vi "Tree.vi"   [LabVIEW 2016, in "Control Experiment.lvclass"]
uses:
  Control Experiment.lvclass
  <userlib>/LevyLab/Krohn Hite 7008/Instrument.KH7008.lvclass
  <userlib>/LevyLab/Lockin-Multichannel/Instrument.Lockin/Instrument.Lockin.lvclass
  <userlib>/LevyLab/LV to ITX/LVtoITX.lvclass
types:
  T1 = typedef "Control Experiment.lvclass/Instruments--cluster.ctl" = cluster{"KH7008":refnum<class "Instrument.KH7008.lvclass">, "Lockin":refnum<class "Instrument.Lockin.lvclass">, "Temperature":refnum<class "Instrument.Cryostat.lvclass">, "Magnet":refnum<class "Instrument.Cryostat.lvclass">, "Rotator":refnum<class "Instrument.Cryostat.lvclass">, "Level":refnum<class "Instrument.Cryostat.lvclass">}
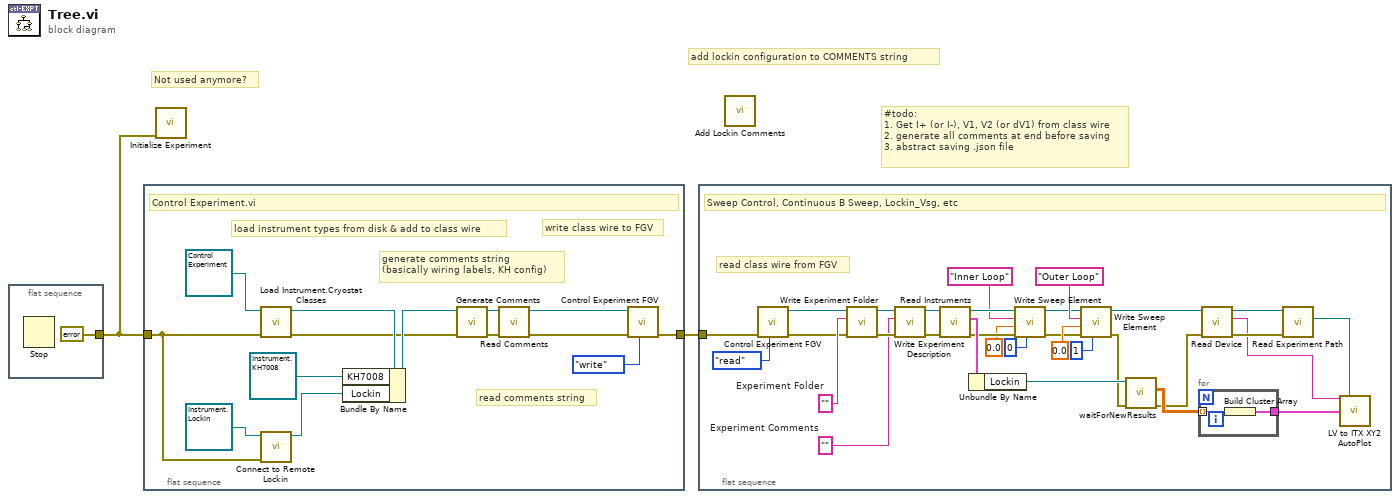
[diagram p0: block diagram]
diagram:
  # "#todo:\n1. Get I+ (or I-), V1, V2 (or dV1) from class wire\n2. generate all comments at end before saving\n3. abstract saving .json file"
  # "add lockin configuration to COMMENTS string"
  # "Not used anymore?"
  n1 = flat-sequence {
    tunnel: [errorcluster {"status"=FALSE, "code"=0, "source"=""} ("error in (no error)")] -> w2
    frame #0 {
      n2 = Stop() -> ()  [unwired: 1 in]
    }
  }
  n3 = flat-sequence {
    tunnel: w2 -> [w5]
    tunnel: [w4] -> w1
    frame #0 {
      # "write class wire to FGV"
      # "read comments string"
      # "generate comments string\n(basically wiring labels, KH config)"
      # "load instrument types from disk & add to class wire"
      # "Control Experiment.vi"
      n4 = call "Load Instrument.Cryostat Classes.vi"("error in (no error)"=w5, "Control Experiment.lvclass"=refnum<class "Control Experiment.lvclass"> refnum) -> ("error out"=w10:errorcluster, "Control Experiment out"=w12:refnum<class "Control Experiment.lvclass">)  [unwired: 8 in]
      n5 = call <userlib>:"Connect to Remote Lockin.vi"("error in (no error)"=w5, "Instrument.Lockin in"=refnum<class "Instrument.Lockin.lvclass"> refnum ("Instruments.Lockin")) -> ("Instrument.Lockin out"=w14:refnum<class "Instrument.Lockin.lvclass">)  [unwired: 8 in, 1 out]
      n6 = Bundle By Name(cluster=w12, "KH7008"=refnum<class "Instrument.KH7008.lvclass"> refnum ("Instruments.KH7008"), "Lockin"=w14) -> (w11:refnum<class "Control Experiment.lvclass">)
      n7 = call "Generate Comments.vi"("error in (no error)"=w10, "Control Experiment"=w11) -> ("error out"=w17:errorcluster, "Control Experiment out"=w16:refnum<class "Control Experiment.lvclass">)  [unwired: 7 in]
      n8 = call "Read Comments.vi"("error in (no error)"=w17, "Control Experiment in"=w16) -> ("error out"=w8:errorcluster, "Control Experiment out"=w7:refnum<class "Control Experiment.lvclass">)  [unwired: 7 in, 1 out]
      n9 = call "Control Experiment FGV.vi"("Function"=enum16{"read", "write"}."write", "error in (no error)"=w8, "Control Experiment.lvclass"=w7) -> ("error out"=w4:errorcluster)  [unwired: 7 in, 1 out]
    }
  }
  n10 = call "Initialize Experiment.vi"("error in (no error)"=w2) -> ()  [unwired: 8 in, 3 out]
  n11 = flat-sequence {
    tunnel: w1 -> [w48]
    frame #0 {
      w43 = ""  # Experiment Comments
      w44 = ""  # Experiment Folder
      # "read class wire from FGV"
      # "Sweep Control, Continuous B Sweep, Lockin_Vsg, etc"
      n12 = call "Control Experiment FGV.vi"("Function"=enum16{"read", "write"}."read", "error in (no error)"=w48) -> ("error out"=w42:errorcluster, "Control Experiment.lvclass out"=w41:refnum<class "Control Experiment.lvclass">)  [unwired: 8 in]
      n13 = call "Write Experiment Folder.vi"("error in (no error)"=w42, "Experiment Folder"=w44, "Control Experiment in"=w41) -> ("error out"=w45:errorcluster, "Control Experiment out"=w46:refnum<class "Control Experiment.lvclass">)  [unwired: 7 in]
      n14 = call "Write Experiment Description.vi"("error in (no error)"=w45, "Experiment Description"=w43, "Control Experiment in"=w46) -> ("error out"=w40:errorcluster, "Control Experiment out"=w39:refnum<class "Control Experiment.lvclass">)  [unwired: 7 in]
      n15 = call "Read Instruments.vi"("error in (no error)"=w40, "Control Experiment in"=w39) -> ("error out"=w31:errorcluster, "Instruments"=w37:T1, "Control Experiment out"=w30:refnum<class "Control Experiment.lvclass">)  [unwired: 7 in]
      n16 = Unbundle By Name(w37) -> ("Lockin"=w36:refnum<class "Instrument.Lockin.lvclass">)
      n17 = call "Write Sweep Element.vi"("loop index"=0, "error in (no error)"=w31, "value"=0.0, "key"="Inner Loop", "Control Experiment in"=w30) -> ("error out"=w21:errorcluster, "Control Experiment out"=w22:refnum<class "Control Experiment.lvclass">)  [unwired: 5 in]
      n18 = call "Write Sweep Element.vi"("loop index"=1, "error in (no error)"=w21, "value"=0.0, "key"="Outer Loop", "Control Experiment in"=w22) -> ("error out"=w19:errorcluster, "Control Experiment out"=w20:refnum<class "Control Experiment.lvclass">)  [unwired: 5 in]
      n19 = call <userlib>:"waitForNewResults.vi"("error in (no error)"=w19, "Instrument.Lockin in"=w36) -> ("error out"=w29:errorcluster, "Results"=w33:dbl[][])  [unwired: 7 in, 1 out]
      n20 = for {
        tunnel: w33 -> [w50] mode=indexing
        tunnel: [w49] -> w32
        n21 = Build Cluster Array(w50) -> (w49:cluster{"Results":dbl[]}[])
      }
      n22 = call "Read Device.vi"("error in (no error)"=w29, "Control Experiment in"=w20) -> ("error out"=w35:errorcluster, "Device"=w18:string, "Control Experiment out"=w38:refnum<class "Control Experiment.lvclass">)  [unwired: 7 in]
      n23 = call "Read Experiment Path.vi"("error in (no error)"=w35, "Control Experiment in"=w38) -> ("Experiment Path"=w34:path)  [unwired: 7 in, 2 out]
      n24 = call <userlib>:"LV to ITX XY2 AutoPlot.vi"("filename"=w18, "path"=w34, "Data"=w32) -> ()  [unwired: 12 in, 1 out]
    }
  }
  n25 = call "Add Lockin Comments.vi"() -> ()  [unwired: 9 in, 2 out]
